vi "Wrong_Address_Multiple_Boards.vi"(1 "In Addresses available":i32[](array[numeric]) format="%x", 2 "numb boards":i32 format="%x") -> (0 "New Address":i32 format="%x")   [LabVIEW 2011]
doc: "This VI is called from \"Start USB\". This is a prompt for the user if none of the USB address of the multiple connected hardware devices matches the address stored in file \"USB_DAQ.ini\"."
panel:
  out "Available Addresses":i32[](array[numeric]) format="%x"
  in  "Current \nSoftware Address":i32 format="%x"
  in  "Abort":bool
  in  "Select New Address\nAnd Press Ok":bool
  in  "Choiose New Address from Available Addresses":u16(ring) items=["2F90", "2F93"]
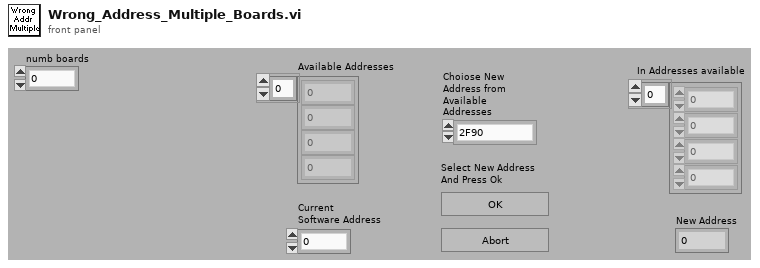
[diagram p1: front panel]
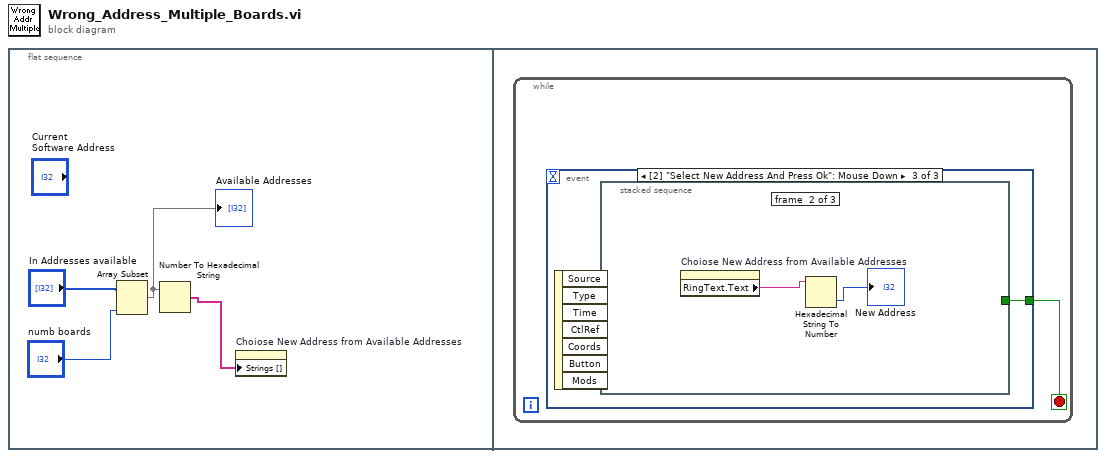
[diagram p0: block diagram]
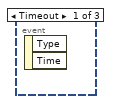
[diagram p2: hidden frame]
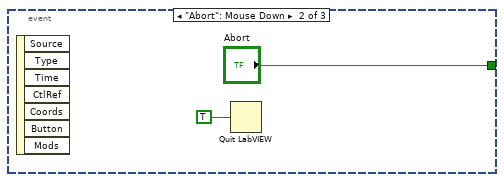
[diagram p3: hidden frame]
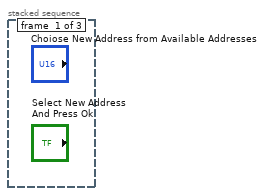
[diagram p4: hidden frame]
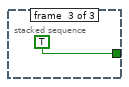
[diagram p5: hidden frame]
diagram:
  n1 = flat-sequence {
    frame #0 {
      n2 = Array Subset(array="In Addresses available", length="numb boards") -> (w1:i32[])  [unwired: 1 in]
      "Available Addresses" <- w1
      n3 = Number To Hexadecimal String(2:w1) -> (0:w4:string[])  [unwired: 1 in]
      n4 = property on="Choiose New Address from Available Addresses" class="Ring (strict)"("Strings []"=w4) -> ()  [unwired: 2 in, 2 out]
    }
    frame #1 {
      n5 = while {
        stop <- w5 stop-if-true
        n6 = event shown="[2] \"Select New Address\nAnd Press Ok\": Mouse Down" {
          selector: _ -> [_ _ _]
          dyn-events: _ -> [_ _ _]
          timeout: _ -> [_ _ _]
          tunnel: [_ "Abort" w8] -> w5
          event Timeout {
            n7 = event-data() -> ()  [unwired: 1 in, 2 out]
          }
          event "Abort": Mouse Down {
            n8 = event-data() -> ()  [unwired: 1 in, 7 out]
            n9 = Quit LabVIEW(quit? (T)=TRUE) -> ()
          }
          event "Select New Address\nAnd Press Ok": Mouse Down {
            n10 = event-data() -> ()  [unwired: 1 in, 7 out]
            n11 = stacked-sequence {
              tunnel: [_ _ TRUE ("quit? (T)")] -> w8
              frame #0 {
              }
              frame #1 {
                n12 = property on="Choiose New Address from Available Addresses" class="Ring (strict)"() -> ("RingText.Text"=w10:string)  [unwired: 2 in, 2 out]
                n13 = Hexadecimal String To Number(string=w10) -> (number=→"New Address":u32)  [unwired: 2 in, 1 out]
              }
              frame #2 {
              }
            }
          }
        }
      }
    }
  }
